vi "Deadband Check.vi"(7 "System Status in":enum16{"Heating", "Cooling", "Idle"}(ring), 8 "error in (no error)":errorcluster, 9 "Cool Setpoint (°F)":dbl, 10 "Hot Setpoint (°F)":dbl, 11 "Current Temperature (°F)":dbl) -> (0 "error out":errorcluster, 5 "System Status out":enum16{"Heating", "Cooling", "Idle"}(ring))   [LabVIEW 2026]
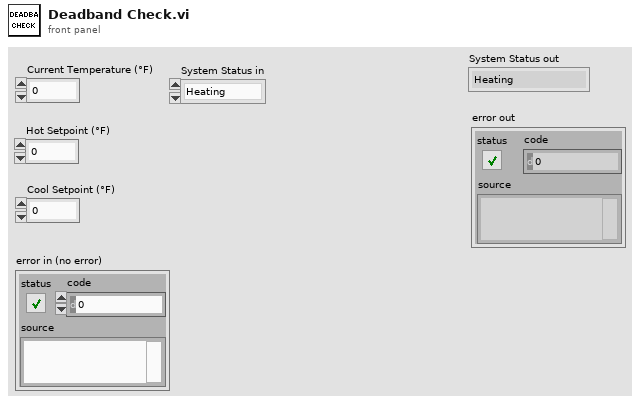
[diagram p1: front panel]
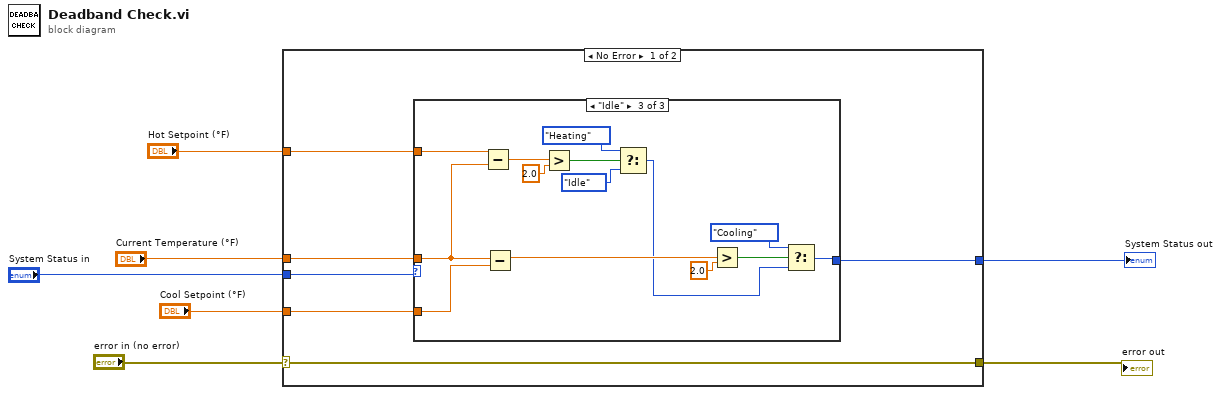
[diagram p0: block diagram]
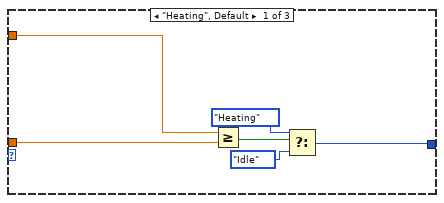
[diagram p2: hidden frame]
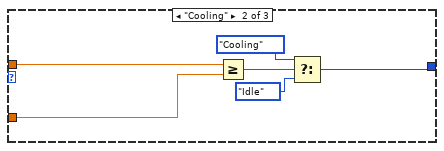
[diagram p3: hidden frame]
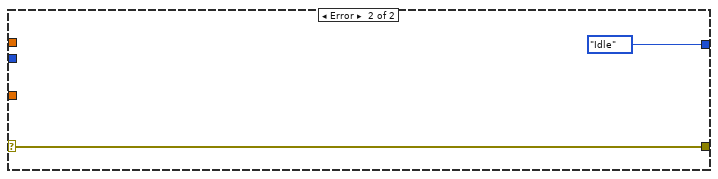
[diagram p4: hidden frame]
diagram:
  n1 = case shown="No Error" "error in (no error)" {
    selector: "error in (no error)" -> [w13 w41]
    tunnel: [w13 w41] -> w6
    tunnel: "Hot Setpoint (°F)" -> [w11 _]
    tunnel: "Cool Setpoint (°F)" -> [w10 _]
    tunnel: "Current Temperature (°F)" -> [w9 _]
    tunnel: "System Status in" -> [w12 _]
    tunnel: [w8 enum16{"Heating", "Cooling", "Idle"}."Idle" ("System Status")] -> w3
    frame No Error {
      n2 = case shown="\"Idle\"" w12 {
        tunnel: w11 -> [w15 _ w34]
        tunnel: w10 -> [_ w20 w38]
        tunnel: w9 -> [w14 w21 w33]
        tunnel: [w16 w22 w26] -> w8
        frame "Heating", Default {
          n3 = Greater Or Equal?(x=w15, y=w14) -> (x >= y?=w19:bool)
          n4 = Select(t=enum16{"Heating", "Cooling", "Idle"}."Heating" ("System Status"), s=w19, f=enum16{"Heating", "Cooling", "Idle"}."Idle" ("System Status")) -> (s? t:f=w16:enum16{"Heating", "Cooling", "Idle"})
        }
        frame "Cooling" {
          n5 = Greater Or Equal?(x=w21, y=w20) -> (x >= y?=w25:bool)
          n6 = Select(t=enum16{"Heating", "Cooling", "Idle"}."Cooling" ("System Status"), s=w25, f=enum16{"Heating", "Cooling", "Idle"}."Idle" ("System Status")) -> (s? t:f=w22:enum16{"Heating", "Cooling", "Idle"})
        }
        frame "Idle" {
          n7 = Subtract(x=w34, y=w33) -> (x-y=w28:dbl)
          n8 = Subtract(x=w33, y=w38) -> (x-y=w39:dbl)
          n9 = Greater?(x=w28, y=2.0) -> (0:w31:bool)
          n10 = Select(t=enum16{"Heating", "Cooling", "Idle"}."Heating" ("System Status"), s=w31, f=enum16{"Heating", "Cooling", "Idle"}."Idle" ("System Status")) -> (s? t:f=w27:enum16{"Heating", "Cooling", "Idle"})
          n11 = Greater?(x=w39, y=2.0) -> (0:w36:bool)
          n12 = Select(t=enum16{"Heating", "Cooling", "Idle"}."Cooling" ("System Status"), s=w36, f=w27) -> (s? t:f=w26:enum16{"Heating", "Cooling", "Idle"})
        }
      }
    }
    frame Error {
    }
  }
  "error out" <- w6
  "System Status out" <- w3
